vi "Create Data File.vi"(0 "DataPath":path, 7 "Test Config":string[](array[string]), 11 "error in":errorcluster) -> (15 "error out":errorcluster)   [LabVIEW 2013]
panel:
  in  "Excel._Application":refnum<k7>
  in  "Excel._Worksheet":refnum<k7>
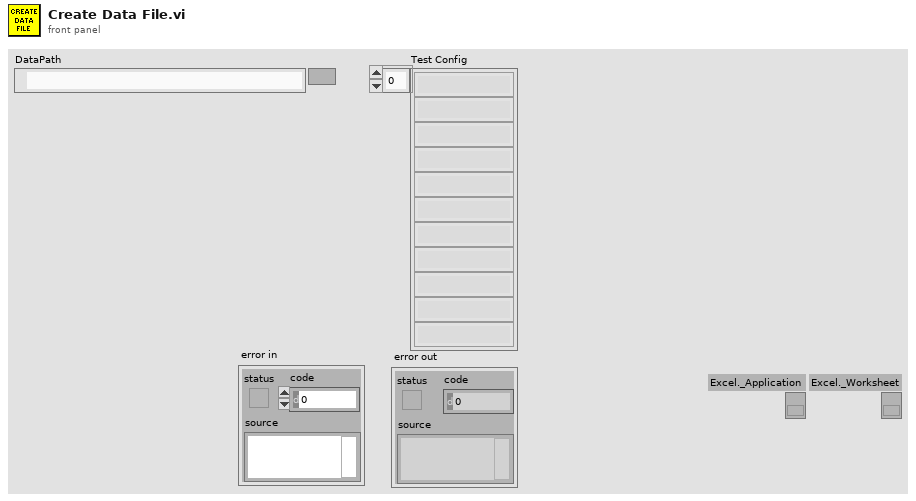
[diagram p1: front panel]
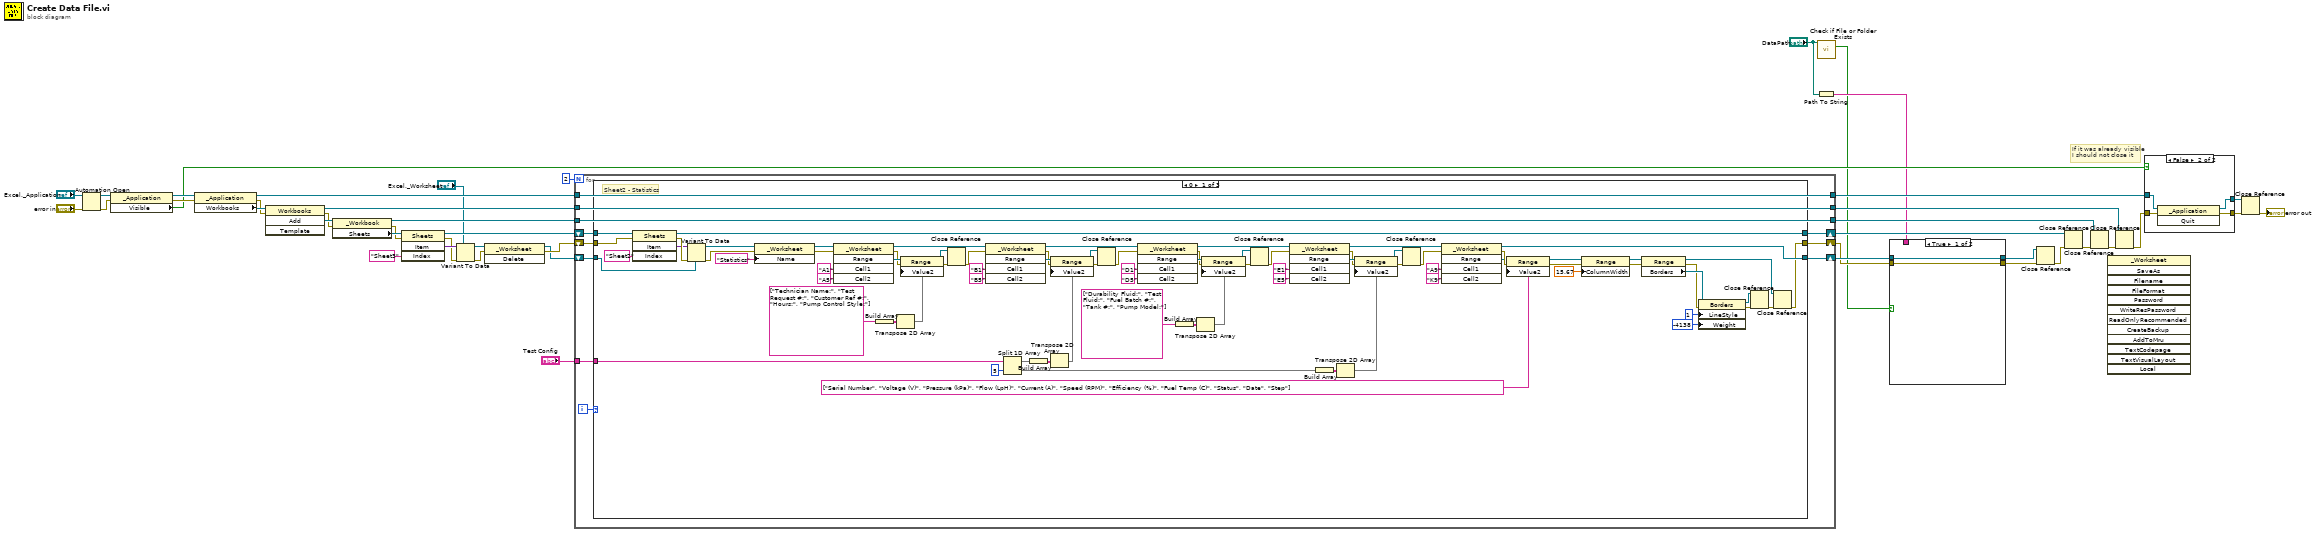
[diagram p0: block diagram]
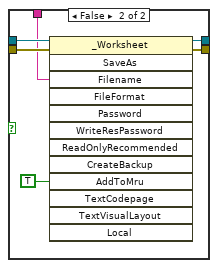
[diagram p2: hidden frame]
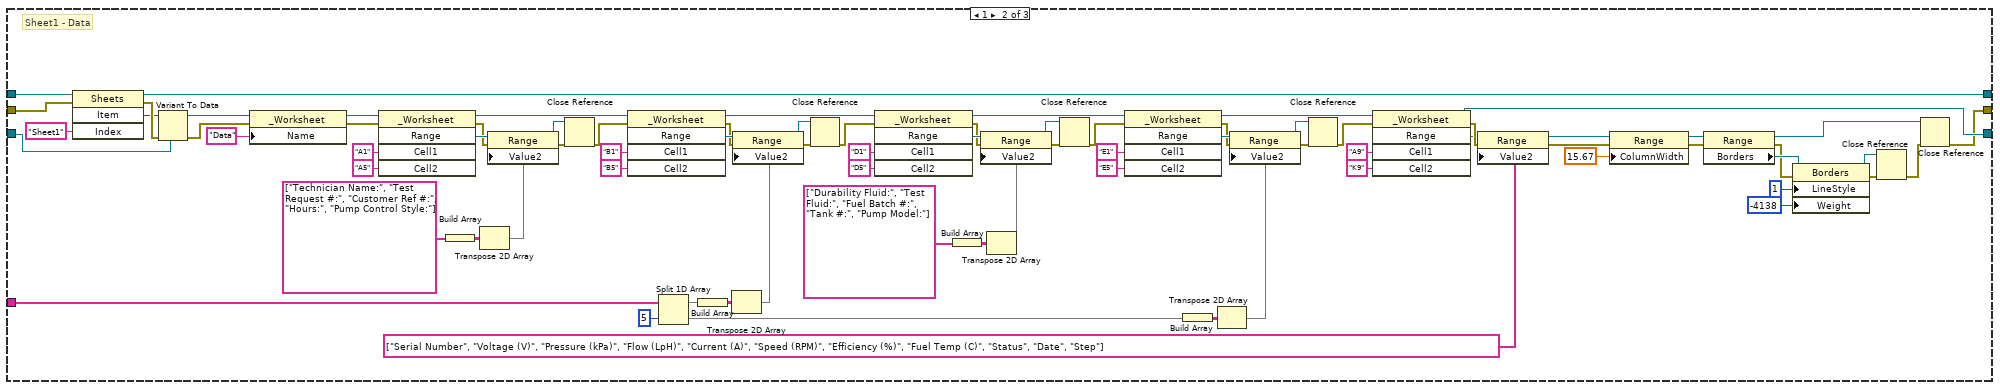
[diagram p4: hidden frame]
diagram:
  # "If it was already visible\nI should not close it"
  n1 = Automation Open(error in (no error)="error in", Automation Refnum="Excel._Application") -> (Automation Refnum=w45:refnum<k7>, error out=w41:errorcluster)  [unwired: 2 in]
  n2 = property class="_Application"(reference=w45, error in=w41) -> (reference out=w44:refnum<k7>, error out=w40:errorcluster, "Visible"=w13:bool)
  n3 = property class="_Application"(reference=w44, error in=w40) -> (reference out=w37:refnum<k7>, error out=w39:errorcluster, "Workbooks"=w43:refnum<k7>)
  n4 = invoke class="Workbooks" method="Add"(reference=w43, error in=w39) -> (reference out=w36:refnum<k7>, error out=w38:errorcluster, "Add"=w42:refnum<k7>)  [unwired: 2 in, 1 out]
  n5 = property class="_Workbook"(reference=w42, error in=w38) -> (reference out=w35:refnum<k7>, error out=w22:errorcluster, "Sheets"=w24:refnum<k7>)
  n6 = invoke class="Sheets" method="Item"(reference=w24, error in=w22, "Index"="Sheet3") -> (reference out=w23:refnum<k7>, error out=w25:errorcluster, "Item"=w26:variant)  [unwired: 1 in, 1 out]
  n7 = Variant To Data(error in=w25, type="Excel._Worksheet", Variant=w26) -> (data=w28:refnum<k7>, error out=w29:errorcluster)
  n8 = invoke class="_Worksheet" method="Delete"(reference=w28, error in=w29) -> (reference out=w10:refnum<k7>, error out=w21:errorcluster)  [unwired: 1 in, 1 out]
  n9 = for {
    N: 2 -> [_]
    tunnel: w37 -> [w50]
    tunnel: w36 -> [w51]
    tunnel: w35 -> [w52]
    shift-right: [w53] -> w7
    shift-left: w21 -> [w54]
    tunnel: [w52] -> w32
    tunnel: [w51] -> w15
    tunnel: [w50] -> w8
    tunnel: "Test Config" -> [w49]
    shift-right: [w48] -> w14
    shift-left: w23 -> [w55]
    shift-right: [w47] -> w9
    shift-left: w10 -> [w46]
    i -> [w56]
    n10 = case shown="0" w56 {
      tunnel: w55 -> [w123 w201 w214]
      tunnel: w54 -> [w122 w200 w215]
      tunnel: [w77 w156 w215] -> w53
      tunnel: w49 -> [w121 w199 _]
      tunnel: [w80 w159 w214] -> w48
      tunnel: [w78 w157 w213] -> w47
      tunnel: w46 -> [w79 w158 w213]
      frame 0 {
        # "Sheet2 - Statistics"
        n11 = invoke class="Sheets" method="Item"(reference=w123, error in=w122, "Index"="Sheet2") -> (reference out=w80:refnum<k7>, error out=w131:errorcluster, "Item"=w130:variant)  [unwired: 1 in, 1 out]
        n12 = Variant To Data(error in=w131, type=w79, Variant=w130) -> (data=w133:refnum<k7>, error out=w132:errorcluster)
        n13 = property class="_Worksheet"(reference=w133, error in=w132, "Name"="Statistics") -> (reference out=w126:refnum<k7>, error out=w128:errorcluster)
        n14 = invoke class="_Worksheet" method="Range"(reference=w126, error in=w128, "Cell1"="A1", "Cell2"="A5") -> (reference out=w110:refnum<k7>, error out=w106:errorcluster, "Range"=w125:refnum<k7>)  [unwired: 1 in, 2 out]
        n15 = Build Array(string[] ["Technician Name:", "Test Request #:", "Customer Ref #:", "Hours:", "Pump Control Style:"]) -> (w68:string[][])
        n16 = Transpose 2D Array(2D array=w68) -> (transposed array=w57:string[][])
        n17 = property class="Range"(reference=w125, error in=w106, "Value2"=w57) -> (reference out=w93:refnum<k7>, error out=w102:errorcluster)
        n18 = Close Reference(reference=w93, error in (no error)=w102) -> (error out=w99:errorcluster)
        n19 = invoke class="_Worksheet" method="Range"(reference=w110, error in=w99, "Cell1"="B1", "Cell2"="B5") -> (reference out=w109:refnum<k7>, error out=w105:errorcluster, "Range"=w118:refnum<k7>)  [unwired: 1 in, 2 out]
        n20 = Split 1D Array(array=w121, index=5) -> (first subarray=w64:string[], second subarray=w61:string[])
        n21 = Build Array(w64) -> (w65:string[][])
        n22 = Transpose 2D Array(2D array=w65) -> (transposed array=w58:string[][])
        n23 = property class="Range"(reference=w118, error in=w105, "Value2"=w58) -> (reference out=w94:refnum<k7>, error out=w101:errorcluster)
        n24 = Close Reference(reference=w94, error in (no error)=w101) -> (error out=w98:errorcluster)
        n25 = invoke class="_Worksheet" method="Range"(reference=w109, error in=w98, "Cell1"="D1", "Cell2"="D5") -> (reference out=w108:refnum<k7>, error out=w104:errorcluster, "Range"=w115:refnum<k7>)  [unwired: 1 in, 2 out]
        n26 = Build Array(string[] ["Durability Fluid:", "Test Fluid:", "Fuel Batch #:", "Tank #:", "Pump Model:"]) -> (w67:string[][])
        n27 = Transpose 2D Array(2D array=w67) -> (transposed array=w59:string[][])
        n28 = property class="Range"(reference=w115, error in=w104, "Value2"=w59) -> (reference out=w95:refnum<k7>, error out=w100:errorcluster)
        n29 = Close Reference(reference=w95, error in (no error)=w100) -> (error out=w97:errorcluster)
        n30 = invoke class="_Worksheet" method="Range"(reference=w108, error in=w97, "Cell1"="E1", "Cell2"="E5") -> (reference out=w87:refnum<k7>, error out=w103:errorcluster, "Range"=w112:refnum<k7>)  [unwired: 1 in, 2 out]
        n31 = Build Array(w61) -> (w66:string[][])
        n32 = Transpose 2D Array(2D array=w66) -> (transposed array=w60:string[][])
        n33 = property class="Range"(reference=w112, error in=w103, "Value2"=w60) -> (reference out=w96:refnum<k7>, error out=w107:errorcluster)
        n34 = Close Reference(reference=w96, error in (no error)=w107) -> (error out=w88:errorcluster)
        n35 = invoke class="_Worksheet" method="Range"(reference=w87, error in=w88, "Cell1"="A9", "Cell2"="K9") -> (reference out=w78:refnum<k7>, error out=w92:errorcluster, "Range"=w90:refnum<k7>)  [unwired: 1 in, 2 out]
        n36 = property class="Range"(reference=w90, error in=w92, "Value2"=string[] ["Serial Number", "Voltage (V)", "Pressure (kPa)", "Flow (LpH)", "Current (A)", "Speed (RPM)", "Efficiency (%)", "Fuel Temp (C)", "Status", "Date", "Step"]) -> (reference out=w73:refnum<k7>, error out=w71:errorcluster)
        n37 = property class="Range"(reference=w73, error in=w71, "ColumnWidth"=15.67) -> (reference out=w69:refnum<k7>, error out=w70:errorcluster)
        n38 = property class="Range"(reference=w69, error in=w70) -> (reference out=w81:refnum<k7>, error out=w76:errorcluster, "Borders"=w85:refnum<k7>)
        n39 = property class="Borders"(reference=w85, error in=w76, "LineStyle"=1, "Weight"=-4138) -> (reference out=w82:refnum<k7>, error out=w84:errorcluster)
        n40 = Close Reference(reference=w82, error in (no error)=w84) -> (error out=w83:errorcluster)
        n41 = Close Reference(reference=w81, error in (no error)=w83) -> (error out=w77:errorcluster)
      }
      frame 1 {
        # "Sheet1 - Data"
        n42 = invoke class="Sheets" method="Item"(reference=w201, error in=w200, "Index"="Sheet1") -> (reference out=w159:refnum<k7>, error out=w209:errorcluster, "Item"=w208:variant)  [unwired: 1 in, 1 out]
        n43 = Variant To Data(error in=w209, type=w158, Variant=w208) -> (data=w211:refnum<k7>, error out=w210:errorcluster)
        n44 = property class="_Worksheet"(reference=w211, error in=w210, "Name"="Data") -> (reference out=w204:refnum<k7>, error out=w206:errorcluster)
        n45 = invoke class="_Worksheet" method="Range"(reference=w204, error in=w206, "Cell1"="A1", "Cell2"="A5") -> (reference out=w188:refnum<k7>, error out=w184:errorcluster, "Range"=w203:refnum<k7>)  [unwired: 1 in, 2 out]
        n46 = Build Array(string[] ["Technician Name:", "Test Request #:", "Customer Ref #:", "Hours:", "Pump Control Style:"]) -> (w154:string[][])
        n47 = Transpose 2D Array(2D array=w154) -> (transposed array=w146:string[][])
        n48 = property class="Range"(reference=w203, error in=w184, "Value2"=w146) -> (reference out=w171:refnum<k7>, error out=w180:errorcluster)
        n49 = Close Reference(reference=w171, error in (no error)=w180) -> (error out=w177:errorcluster)
        n50 = invoke class="_Worksheet" method="Range"(reference=w188, error in=w177, "Cell1"="B1", "Cell2"="B5") -> (reference out=w187:refnum<k7>, error out=w183:errorcluster, "Range"=w196:refnum<k7>)  [unwired: 1 in, 2 out]
        n51 = Split 1D Array(array=w199, index=5) -> (first subarray=w148:string[], second subarray=w150:string[])
        n52 = Build Array(w148) -> (w153:string[][])
        n53 = Transpose 2D Array(2D array=w153) -> (transposed array=w145:string[][])
        n54 = property class="Range"(reference=w196, error in=w183, "Value2"=w145) -> (reference out=w172:refnum<k7>, error out=w179:errorcluster)
        n55 = Close Reference(reference=w172, error in (no error)=w179) -> (error out=w176:errorcluster)
        n56 = invoke class="_Worksheet" method="Range"(reference=w187, error in=w176, "Cell1"="D1", "Cell2"="D5") -> (reference out=w186:refnum<k7>, error out=w182:errorcluster, "Range"=w193:refnum<k7>)  [unwired: 1 in, 2 out]
        n57 = Build Array(string[] ["Durability Fluid:", "Test Fluid:", "Fuel Batch #:", "Tank #:", "Pump Model:"]) -> (w152:string[][])
        n58 = Transpose 2D Array(2D array=w152) -> (transposed array=w144:string[][])
        n59 = property class="Range"(reference=w193, error in=w182, "Value2"=w144) -> (reference out=w173:refnum<k7>, error out=w178:errorcluster)
        n60 = Close Reference(reference=w173, error in (no error)=w178) -> (error out=w175:errorcluster)
        n61 = invoke class="_Worksheet" method="Range"(reference=w186, error in=w175, "Cell1"="E1", "Cell2"="E5") -> (reference out=w165:refnum<k7>, error out=w181:errorcluster, "Range"=w190:refnum<k7>)  [unwired: 1 in, 2 out]
        n62 = Build Array(w150) -> (w151:string[][])
        n63 = Transpose 2D Array(2D array=w151) -> (transposed array=w143:string[][])
        n64 = property class="Range"(reference=w190, error in=w181, "Value2"=w143) -> (reference out=w174:refnum<k7>, error out=w185:errorcluster)
        n65 = Close Reference(reference=w174, error in (no error)=w185) -> (error out=w166:errorcluster)
        n66 = invoke class="_Worksheet" method="Range"(reference=w165, error in=w166, "Cell1"="A9", "Cell2"="K9") -> (reference out=w157:refnum<k7>, error out=w170:errorcluster, "Range"=w168:refnum<k7>)  [unwired: 1 in, 2 out]
        n67 = property class="Range"(reference=w168, error in=w170, "Value2"=string[] ["Serial Number", "Voltage (V)", "Pressure (kPa)", "Flow (LpH)", "Current (A)", "Speed (RPM)", "Efficiency (%)", "Fuel Temp (C)", "Status", "Date", "Step"]) -> (reference out=w138:refnum<k7>, error out=w137:errorcluster)
        n68 = property class="Range"(reference=w138, error in=w137, "ColumnWidth"=15.67) -> (reference out=w135:refnum<k7>, error out=w136:errorcluster)
        n69 = property class="Range"(reference=w135, error in=w136) -> (reference out=w160:refnum<k7>, error out=w155:errorcluster, "Borders"=w164:refnum<k7>)
        n70 = property class="Borders"(reference=w164, error in=w155, "LineStyle"=1, "Weight"=-4138) -> (reference out=w162:refnum<k7>, error out=w163:errorcluster)
        n71 = Close Reference(reference=w162, error in (no error)=w163) -> (error out=w161:errorcluster)
        n72 = Close Reference(reference=w160, error in (no error)=w161) -> (error out=w156:errorcluster)
      }
      frame Default {
      }
    }
  }
  n73 = Path To String(path="DataPath") -> (string=w2:string)
  n74 = call <vilib>:"Check if File or Folder Exists.vi"("path"="DataPath") -> ("file or folder exists?"=w1:bool)  [unwired: 8 in, 2 out]
  n75 = case shown="True" w1 {
    tunnel: w9 -> [w217 w223]
    tunnel: w7 -> [w216 w221]
    tunnel: [w217 w220] -> w6
    tunnel: [w216 w219] -> w5
    tunnel: w2 -> [_ w218]
    frame True {
    }
    frame False {
      n76 = invoke class="_Worksheet" method="SaveAs"(reference=w223, error in=w221, "Filename"=w218, "AddToMru"=TRUE) -> (reference out=w220:refnum<k7>, error out=w219:errorcluster)  [unwired: 9 in, 11 out]
    }
  }
  n77 = Close Reference(reference=w6, error in (no error)=w5) -> (error out=w20:errorcluster)
  n78 = Close Reference(reference=w14, error in (no error)=w20) -> (error out=w30:errorcluster)
  n79 = Close Reference(reference=w32, error in (no error)=w30) -> (error out=w33:errorcluster)
  n80 = invoke class="_Worksheet" method="SaveAs"() -> ()  [unwired: 13 in, 13 out]
  n81 = Close Reference(reference=w15, error in (no error)=w33) -> (error out=w4:errorcluster)
  n82 = case shown="False" w13 {
    tunnel: w8 -> [w225 w229]
    tunnel: w4 -> [w224 w228]
    tunnel: [w225 w227] -> w11
    tunnel: [w224 w226] -> w12
    frame True {
    }
    frame False {
      n83 = invoke class="_Application" method="Quit"(reference=w229, error in=w228) -> (reference out=w227:refnum<k7>, error out=w226:errorcluster)  [unwired: 1 in, 1 out]
    }
  }
  n84 = Close Reference(reference=w11, error in (no error)=w12) -> (error out=→"error out":errorcluster)
